vi "Convert Ref Value To Class.vi"(8 "error in (no error)":errorcluster, 10 "Main Ctls and VI Refs":refnum<vi>[](array[refnum]), 11 "MemberInfo in":refnum<class "Information.lvclass">) -> (0 "error out":errorcluster, 3 "MemberInfo out":refnum<class "Information.lvclass">)   [LabVIEW 2015, in "Information.lvclass"]
uses:
  Information.lvclass
  Type Definitions/UserInfo.ctl
  Information.lvclass/Information.ctl
panel:
  in  "UserInfo":T1
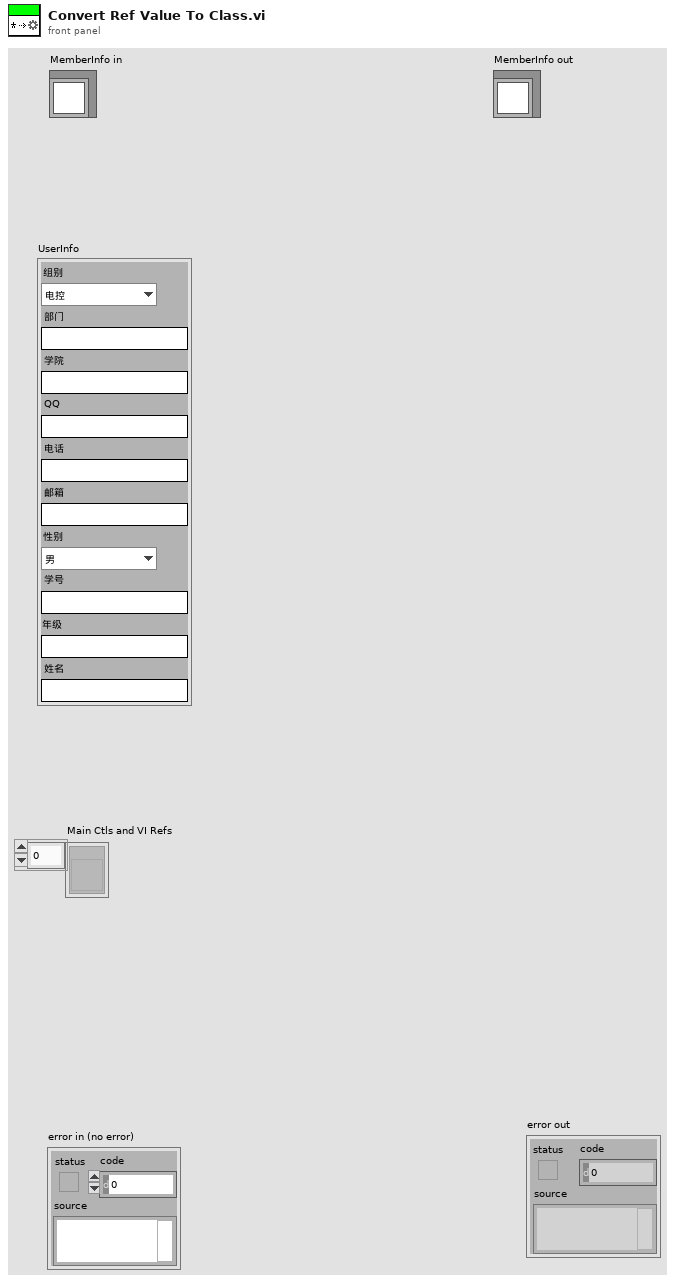
[diagram p1: front panel]
types:
  T1 = typedef "Information.lvclass/UserInfo.ctl" = cluster{"组别":enum16{"电控", "机械", "视觉"}, "部门":string, "学院":string, "QQ":string, "电话":string, "邮箱":string, "性别":enum16{"男", "女"}, "学号":string, "年级":string, "姓名":string}
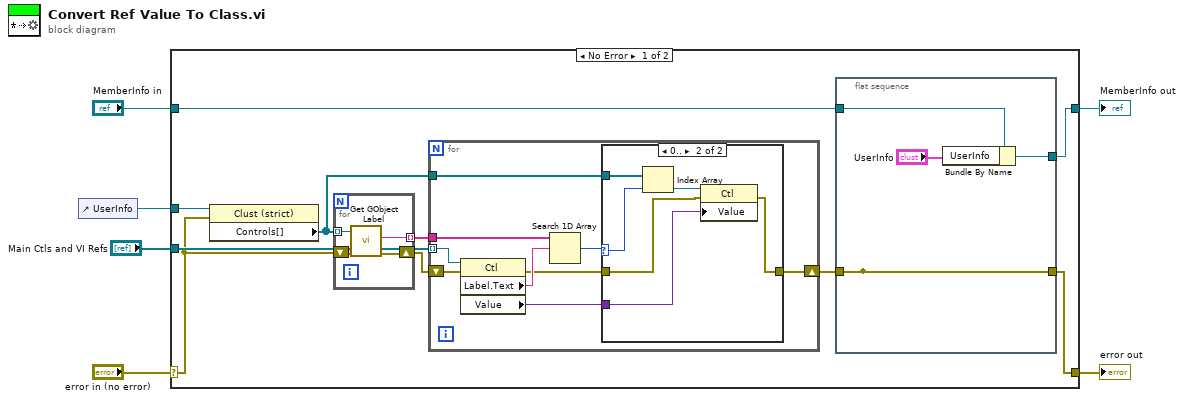
[diagram p0: block diagram]
diagram:
  n1 = control-ref of="UserInfo"() -> (w1:refnum<vi>)
  n2 = case shown="No Error" "error in (no error)" {
    selector: "error in (no error)" -> [w14 w42]
    tunnel: [w7 w42] -> w5
    tunnel: [w8 w41] -> w3
    tunnel: "MemberInfo in" -> [w9 w41]
    tunnel: "Main Ctls and VI Refs" -> [w16 _]
    tunnel: w1 -> [w15 _]
    frame No Error {
      n3 = property class="Clust (strict)"(reference=w15, error in=w14) -> ("Controls[]"=w11:refnum<vi>[])  [unwired: 2 out]
      n4 = for {
        tunnel: w11 -> [w24] mode=indexing
        tunnel: [w22] -> w12 mode=indexing
        shift-right: [w21] -> w13
        shift-left: w14 -> [w23]
        n5 = call <vilib>:"Get GObject Label.vi"("error in (no error)"=w23, "GObject"=w24) -> ("error out"=w21:errorcluster, "Object Label"=w22:string)  [unwired: 5 in, 3 out]
      }
      n6 = for {
        tunnel: w16 -> [w33] mode=indexing
        tunnel: w12 -> [w31]
        tunnel: w11 -> [w28]
        shift-right: [w25] -> w10
        shift-left: w13 -> [w32]
        n7 = property class="Ctl"(reference=w33, error in=w32) -> (error out=w26:errorcluster, "Label.Text"=w30:string, "Value"=w27:variant)  [unwired: 1 out]
        n8 = Search 1D Array(1D array=w31, element=w30) -> (index of element=w29:i32)  [unwired: 1 in]
        n9 = case shown="0.." w29 {
          selector: w29 -> [_ w39]
          tunnel: w28 -> [_ w40]
          tunnel: w27 -> [_ w37]
          tunnel: w26 -> [w34 w36]
          tunnel: [w34 w35] -> w25
          frame Default {
          }
          frame 0.. {
            n10 = Index Array(array=w40, index=w39) -> (element=w38:refnum<vi>)
            n11 = property class="Ctl"(reference=w38, error in=w36, "Value"=w37) -> (error out=w35:errorcluster)  [unwired: 1 out]
          }
        }
      }
      n12 = flat-sequence {
        tunnel: w10 -> [w17]
        tunnel: w9 -> [w20]
        tunnel: [w18] -> w8
        tunnel: [w17] -> _
        tunnel: [w17] -> w7
        frame #0 {
          n13 = Bundle By Name(cluster=w20, "UserInfo"="UserInfo") -> (w18:refnum<class "Information.lvclass">)
        }
      }
    }
    frame Error {
    }
  }
  "error out" <- w5
  "MemberInfo out" <- w3
